vi "FL_Calc_speed_on_the_fly.vi"(1 "Y coord, mm":dbl, 2 "X coord, mm":dbl, 3 "Time per frame, s":dbl) -> (0 "Mouse speed, mm/s":dbl)   [LabVIEW 2016]
doc: "This VI calculates speed using smoothing of the input noisy data according to Holoborodko' algorithm: http://www.holoborodko.com/pavel/numerical-methods/numerical-derivative/smooth-low-noise-differentiator"
uses:
  <vilib>/Analysis/baseanly.llb/Mean (DBL).vi
  <vilib>/Analysis/NI_AALBase.lvlib
panel:
  in  "Speed smoothing type":u16(ring)=3 items=["None", "Holoborodko 2/5", "Holoborodko 2/7", "Holoborodko 2/11", "Holoborodko 4/7"]
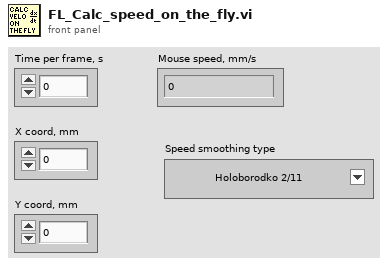
[diagram p1: front panel]
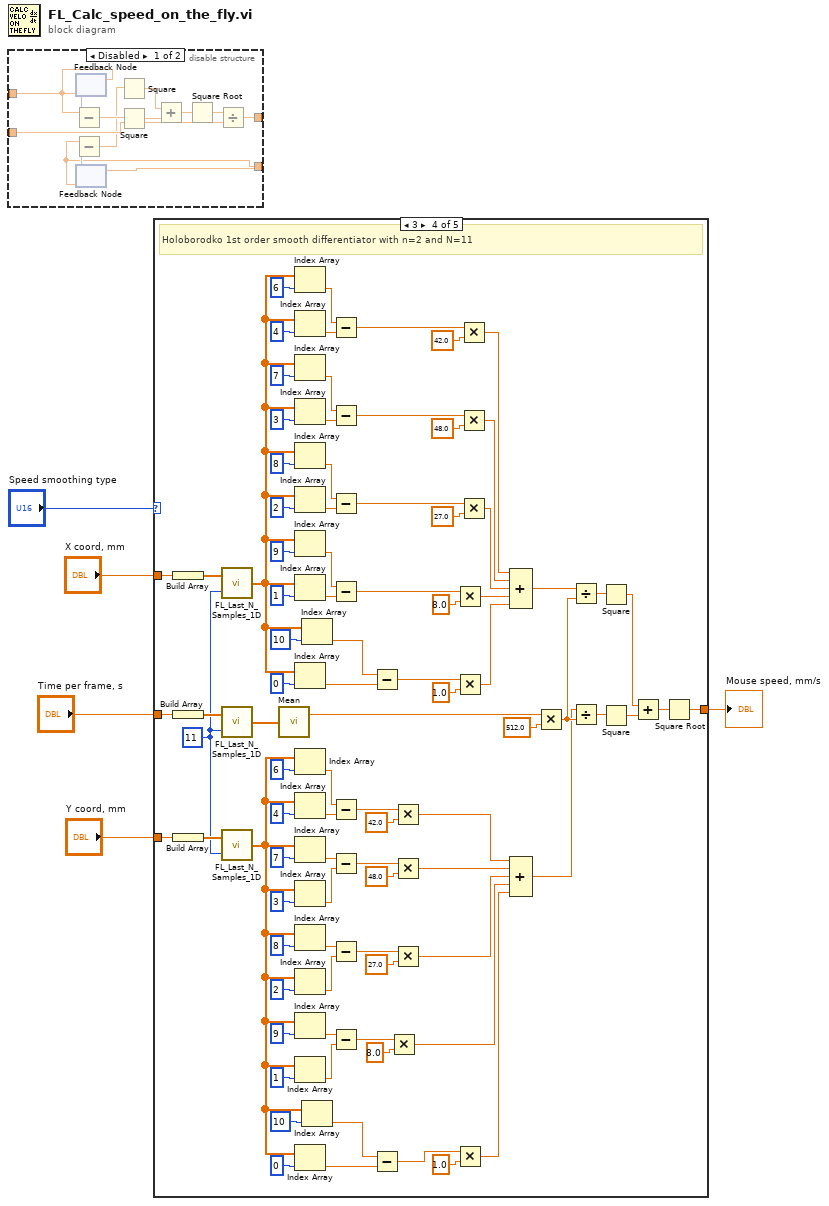
[diagram p0: block diagram]
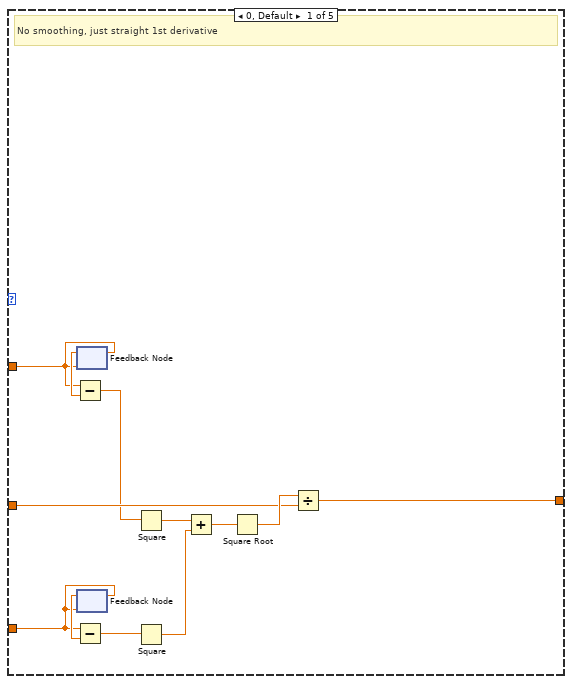
[diagram p2: hidden frame]
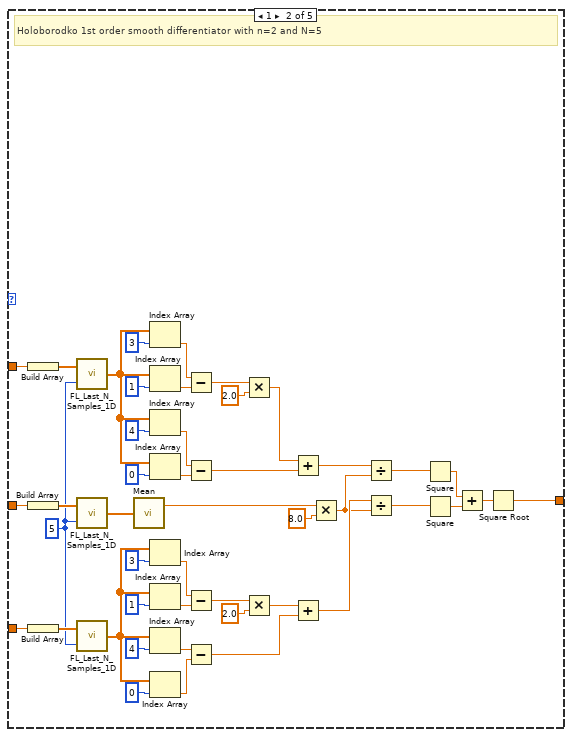
[diagram p3: hidden frame]
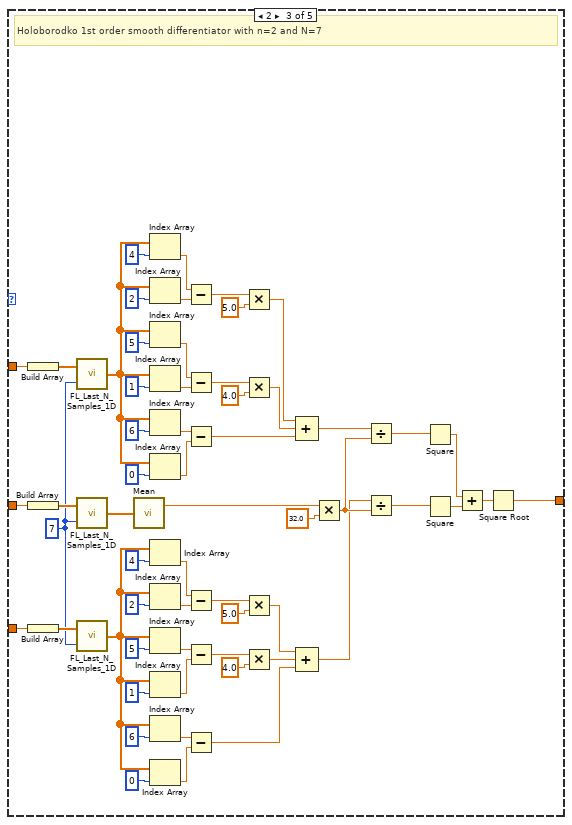
[diagram p4: hidden frame]
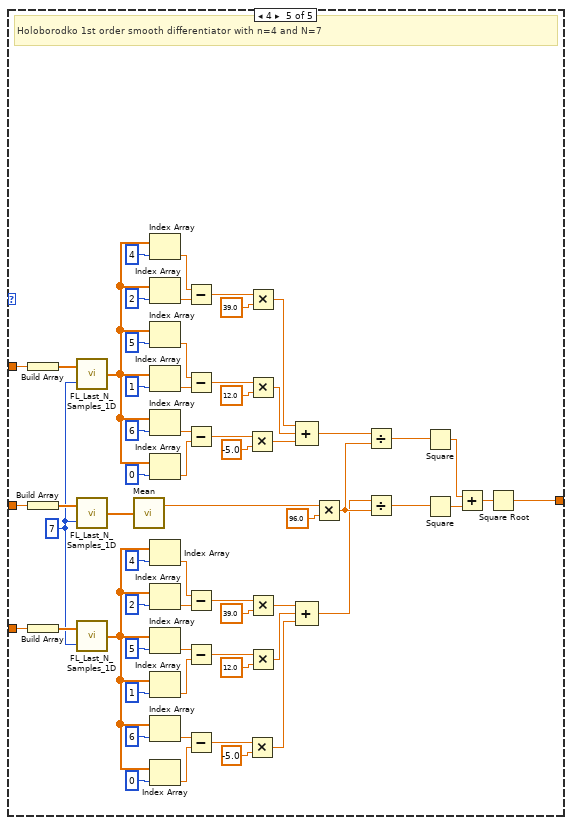
[diagram p5: hidden frame]
diagram:
  n1 = disable-structure shown="Disabled" {
    disable-tunnel: _ -> [w17 _]
    disable-tunnel: [w16 _] -> _
    disable-tunnel: _ -> [w15 _]
    disable-tunnel: _ -> [w6 _]
    frame Disabled {
      n2 = feedback #1(w15) -> (w8)
      n3 = Subtract(x=w15, y=w8) -> (x-y=w10:dbl)
      n4 = feedback-in #1(w15) -> ()
      n5 = feedback #2(w6) -> (w7)
      n6 = Subtract(x=w6, y=w7) -> (x-y=w9:dbl)
      n7 = feedback-in #2(w6) -> ()
      n8 = Square(x=w9) -> (x^2=w12:dbl)
      n9 = Square(x=w10) -> (x^2=w11:dbl)
      n10 = Add(x=w12, y=w11) -> (x+y=w13:dbl)
      n11 = Square Root(x=w13) -> (sqrt(x)=w14:dbl)
      n12 = Divide(x=w14, y=w17) -> (x/y=w16:dbl)
    }
    frame Enabled {
    }
  }
  n13 = case shown="3" "Speed smoothing type" {
    tunnel: "Time per frame, s" -> [w25 w74 w133 w224 w287]
    tunnel: "Y coord, mm" -> [w19 w70 w129 w220 w283]
    tunnel: "X coord, mm" -> [w21 w69 w128 w219 w282]
    tunnel: [w24 w30 w109 w200 w263] -> w2
    frame 0, Default {
      # "No smoothing, just straight 1st derivative"
      n14 = feedback #3(w21) -> (w22:dbl)
      n15 = Subtract(x=w21, y=w22) -> (x-y=w20:dbl)
      n16 = feedback-in #3(w21) -> ()
      n17 = feedback #4(w19) -> (w23:dbl)
      n18 = Subtract(x=w19, y=w23) -> (x-y=w18:dbl)
      n19 = feedback-in #4(w19) -> ()
      n20 = Square(x=w20) -> (x^2=w28:dbl)
      n21 = Square(x=w18) -> (x^2=w29:dbl)
      n22 = Add(x=w28, y=w29) -> (x+y=w27:dbl)
      n23 = Square Root(x=w27) -> (sqrt(x)=w26:dbl)
      n24 = Divide(x=w26, y=w25) -> (x/y=w24:dbl)
    }
    frame 1 {
      w68 = u32 5 ("BufferLengthSamples")
      # "Holoborodko 1st order smooth differentiator with n=2 and N=5"
      n25 = Build Array(w69) -> (w72:dbl[])
      n26 = Build Array(w74) -> (w73:dbl[])
      n27 = Build Array(w70) -> (w71:dbl[])
      n28 = call "FL_Last_N_Samples_1D.vi"("BufferLengthSamples"=w68, "Input Array of strings"=w72) -> ("Output Array of strings"=w58:dbl[])
      n29 = call "FL_Last_N_Samples_1D.vi"("BufferLengthSamples"=w68, "Input Array of strings"=w73) -> ("Output Array of strings"=w67:dbl[])
      n30 = call "FL_Last_N_Samples_1D.vi"("BufferLengthSamples"=w68, "Input Array of strings"=w71) -> ("Output Array of strings"=w37:dbl[])
      n31 = call-poly <vilib>:"Mean.vi"("X"=w67) -> ("mean"=w52:dbl)  [unwired: 1 out]
      n32 = Index Array(array=w58, index=3) -> (element=w64:dbl)
      n33 = Index Array(array=w58, index=1) -> (element=w63:dbl)
      n34 = Index Array(array=w58, index=4) -> (element=w57:dbl)
      n35 = Index Array(array=w58, index=0) -> (element=w56:dbl)
      n36 = Index Array(array=w37, index=3) -> (element=w40:dbl)
      n37 = Index Array(array=w37, index=1) -> (element=w41:dbl)
      n38 = Index Array(array=w37, index=4) -> (element=w46:dbl)
      n39 = Index Array(array=w37, index=0) -> (element=w47:dbl)
      n40 = Subtract(x=w64, y=w63) -> (x-y=w62:dbl)
      n41 = Subtract(x=w57, y=w56) -> (x-y=w54:dbl)
      n42 = Subtract(x=w40, y=w41) -> (x-y=w42:dbl)
      n43 = Subtract(x=w46, y=w47) -> (x-y=w49:dbl)
      n44 = Multiply(x=w62, y=2.0) -> (x*y=w55:dbl)
      n45 = Multiply(x=w42, y=2.0) -> (x*y=w48:dbl)
      n46 = Add(x=w55, y=w54) -> (x+y=w53:dbl)
      n47 = Add(x=w48, y=w49) -> (x+y=w50:dbl)
      n48 = Multiply(x=w52, y=8.0) -> (x*y=w36:dbl)
      n49 = Divide(x=w53, y=w36) -> (x/y=w33:dbl)
      n50 = Divide(x=w50, y=w36) -> (x/y=w31:dbl)
      n51 = Square(x=w33) -> (x^2=w32:dbl)
      n52 = Square(x=w31) -> (x^2=w34:dbl)
      n53 = Add(x=w32, y=w34) -> (x+y=w35:dbl)
      n54 = Square Root(x=w35) -> (sqrt(x)=w30:dbl)
    }
    frame 2 {
      w127 = u32 7 ("BufferLengthSamples")
      # "Holoborodko 1st order smooth differentiator with n=2 and N=7"
      n55 = Build Array(w128) -> (w131:dbl[])
      n56 = Build Array(w133) -> (w132:dbl[])
      n57 = Build Array(w129) -> (w130:dbl[])
      n58 = call "FL_Last_N_Samples_1D.vi"("BufferLengthSamples"=w127, "Input Array of strings"=w131) -> ("Output Array of strings"=w104:dbl[])
      n59 = call "FL_Last_N_Samples_1D.vi"("BufferLengthSamples"=w127, "Input Array of strings"=w132) -> ("Output Array of strings"=w126:dbl[])
      n60 = call "FL_Last_N_Samples_1D.vi"("BufferLengthSamples"=w127, "Input Array of strings"=w130) -> ("Output Array of strings"=w77:dbl[])
      n61 = call-poly <vilib>:"Mean.vi"("X"=w126) -> ("mean"=w117:dbl)  [unwired: 1 out]
      n62 = Index Array(array=w104, index=4) -> (element=w123:dbl)
      n63 = Index Array(array=w104, index=2) -> (element=w122:dbl)
      n64 = Index Array(array=w104, index=5) -> (element=w119:dbl)
      n65 = Index Array(array=w104, index=1) -> (element=w118:dbl)
      n66 = Index Array(array=w104, index=6) -> (element=w107:dbl)
      n67 = Index Array(array=w104, index=0) -> (element=w108:dbl)
      n68 = Index Array(array=w77, index=4) -> (element=w80:dbl)
      n69 = Index Array(array=w77, index=2) -> (element=w81:dbl)
      n70 = Index Array(array=w77, index=5) -> (element=w84:dbl)
      n71 = Index Array(array=w77, index=1) -> (element=w85:dbl)
      n72 = Index Array(array=w77, index=6) -> (element=w87:dbl)
      n73 = Index Array(array=w77, index=0) -> (element=w86:dbl)
      n74 = Subtract(x=w123, y=w122) -> (x-y=w103:dbl)
      n75 = Subtract(x=w119, y=w118) -> (x-y=w101:dbl)
      n76 = Subtract(x=w107, y=w108) -> (x-y=w99:dbl)
      n77 = Subtract(x=w80, y=w81) -> (x-y=w90:dbl)
      n78 = Subtract(x=w84, y=w85) -> (x-y=w92:dbl)
      n79 = Subtract(x=w87, y=w86) -> (x-y=w94:dbl)
      n80 = Multiply(x=w103, y=5.0) -> (x*y=w97:dbl)
      n81 = Multiply(x=w101, y=4.0) -> (x*y=w98:dbl)
      n82 = Multiply(x=w90, y=5.0) -> (x*y=w96:dbl)
      n83 = Multiply(x=w92, y=4.0) -> (x*y=w95:dbl)
      n84 = Compound Arithmetic op=ADD(w97, w98, w99) -> (w76:dbl)
      n85 = Compound Arithmetic op=ADD(w96, w95, w94) -> (w75:dbl)
      n86 = Multiply(x=w117, y=32.0) -> (x*y=w115:dbl)
      n87 = Divide(x=w76, y=w115) -> (x/y=w112:dbl)
      n88 = Divide(x=w75, y=w115) -> (x/y=w110:dbl)
      n89 = Square(x=w112) -> (x^2=w111:dbl)
      n90 = Square(x=w110) -> (x^2=w113:dbl)
      n91 = Add(x=w111, y=w113) -> (x+y=w114:dbl)
      n92 = Square Root(x=w114) -> (sqrt(x)=w109:dbl)
    }
    frame 3 {
      w218 = u32 11 ("BufferLengthSamples")
      # "Holoborodko 1st order smooth differentiator with n=2 and N=11"
      n93 = Build Array(w219) -> (w222:dbl[])
      n94 = Build Array(w224) -> (w223:dbl[])
      n95 = Build Array(w220) -> (w221:dbl[])
      n96 = call "FL_Last_N_Samples_1D.vi"("BufferLengthSamples"=w218, "Input Array of strings"=w222) -> ("Output Array of strings"=w173:dbl[])
      n97 = call "FL_Last_N_Samples_1D.vi"("BufferLengthSamples"=w218, "Input Array of strings"=w223) -> ("Output Array of strings"=w217:dbl[])
      n98 = call "FL_Last_N_Samples_1D.vi"("BufferLengthSamples"=w218, "Input Array of strings"=w221) -> ("Output Array of strings"=w135:dbl[])
      n99 = call-poly <vilib>:"Mean.vi"("X"=w217) -> ("mean"=w208:dbl)  [unwired: 1 out]
      n100 = Index Array(array=w173, index=6) -> (element=w214:dbl)
      n101 = Index Array(array=w173, index=4) -> (element=w213:dbl)
      n102 = Index Array(array=w173, index=7) -> (element=w210:dbl)
      n103 = Index Array(array=w173, index=3) -> (element=w209:dbl)
      n104 = Index Array(array=w173, index=8) -> (element=w198:dbl)
      n105 = Index Array(array=w173, index=2) -> (element=w199:dbl)
      n106 = Index Array(array=w173, index=9) -> (element=w181:dbl)
      n107 = Index Array(array=w173, index=1) -> (element=w180:dbl)
      n108 = Index Array(array=w173, index=0) -> (element=w179:dbl)
      n109 = Index Array(array=w135, index=6) -> (element=w138:dbl)
      n110 = Index Array(array=w135, index=4) -> (element=w139:dbl)
      n111 = Index Array(array=w135, index=7) -> (element=w142:dbl)
      n112 = Index Array(array=w135, index=3) -> (element=w143:dbl)
      n113 = Index Array(array=w135, index=8) -> (element=w145:dbl)
      n114 = Index Array(array=w135, index=2) -> (element=w144:dbl)
      n115 = Index Array(array=w135, index=9) -> (element=w161:dbl)
      n116 = Index Array(array=w135, index=1) -> (element=w162:dbl)
      n117 = Index Array(array=w135, index=0) -> (element=w163:dbl)
      n118 = Index Array(array=w173, index=10) -> (element=w178:dbl)
      n119 = Index Array(array=w135, index=10) -> (element=w164:dbl)
      n120 = Subtract(x=w214, y=w213) -> (x-y=w195:dbl)
      n121 = Subtract(x=w210, y=w209) -> (x-y=w193:dbl)
      n122 = Subtract(x=w198, y=w199) -> (x-y=w191:dbl)
      n123 = Subtract(x=w181, y=w180) -> (x-y=w184:dbl)
      n124 = Subtract(x=w138, y=w139) -> (x-y=w148:dbl)
      n125 = Subtract(x=w142, y=w143) -> (x-y=w150:dbl)
      n126 = Subtract(x=w145, y=w144) -> (x-y=w152:dbl)
      n127 = Subtract(x=w161, y=w162) -> (x-y=w158:dbl)
      n128 = Subtract(x=w178, y=w179) -> (x-y=w175:dbl)
      n129 = Subtract(x=w164, y=w163) -> (x-y=w167:dbl)
      n130 = Multiply(x=w158, y=8.0) -> (x*y=w169:dbl)
      n131 = Multiply(x=w148, y=42.0) -> (x*y=w154:dbl)
      n132 = Multiply(x=w150, y=48.0) -> (x*y=w153:dbl)
      n133 = Multiply(x=w152, y=27.0) -> (x*y=w155:dbl)
      n134 = Multiply(x=w184, y=8.0) -> (x*y=w172:dbl)
      n135 = Multiply(x=w175, y=1.0) -> (x*y=w171:dbl)
      n136 = Multiply(x=w167, y=1.0) -> (x*y=w170:dbl)
      n137 = Multiply(x=w195, y=42.0) -> (x*y=w189:dbl)
      n138 = Multiply(x=w193, y=48.0) -> (x*y=w190:dbl)
      n139 = Multiply(x=w191, y=27.0) -> (x*y=w187:dbl)
      n140 = Compound Arithmetic op=ADD(w189, w190, w187, w172, w171) -> (w188:dbl)
      n141 = Compound Arithmetic op=ADD(w154, w153, w155, w169, w170) -> (w134:dbl)
      n142 = Multiply(x=w208, y=512.0) -> (x*y=w206:dbl)
      n143 = Divide(x=w188, y=w206) -> (x/y=w203:dbl)
      n144 = Divide(x=w134, y=w206) -> (x/y=w201:dbl)
      n145 = Square(x=w203) -> (x^2=w202:dbl)
      n146 = Square(x=w201) -> (x^2=w204:dbl)
      n147 = Add(x=w202, y=w204) -> (x+y=w205:dbl)
      n148 = Square Root(x=w205) -> (sqrt(x)=w200:dbl)
    }
    frame 4 {
      w281 = u32 7 ("BufferLengthSamples")
      # "Holoborodko 1st order smooth differentiator with n=4 and N=7"
      n149 = Build Array(w282) -> (w285:dbl[])
      n150 = Build Array(w287) -> (w286:dbl[])
      n151 = Build Array(w283) -> (w284:dbl[])
      n152 = call "FL_Last_N_Samples_1D.vi"("BufferLengthSamples"=w281, "Input Array of strings"=w285) -> ("Output Array of strings"=w258:dbl[])
      n153 = call "FL_Last_N_Samples_1D.vi"("BufferLengthSamples"=w281, "Input Array of strings"=w286) -> ("Output Array of strings"=w280:dbl[])
      n154 = call "FL_Last_N_Samples_1D.vi"("BufferLengthSamples"=w281, "Input Array of strings"=w284) -> ("Output Array of strings"=w231:dbl[])
      n155 = call-poly <vilib>:"Mean.vi"("X"=w280) -> ("mean"=w271:dbl)  [unwired: 1 out]
      n156 = Index Array(array=w258, index=4) -> (element=w277:dbl)
      n157 = Index Array(array=w258, index=2) -> (element=w276:dbl)
      n158 = Index Array(array=w258, index=5) -> (element=w273:dbl)
      n159 = Index Array(array=w258, index=1) -> (element=w272:dbl)
      n160 = Index Array(array=w258, index=6) -> (element=w261:dbl)
      n161 = Index Array(array=w258, index=0) -> (element=w262:dbl)
      n162 = Index Array(array=w231, index=4) -> (element=w234:dbl)
      n163 = Index Array(array=w231, index=2) -> (element=w235:dbl)
      n164 = Index Array(array=w231, index=5) -> (element=w238:dbl)
      n165 = Index Array(array=w231, index=1) -> (element=w239:dbl)
      n166 = Index Array(array=w231, index=6) -> (element=w241:dbl)
      n167 = Index Array(array=w231, index=0) -> (element=w240:dbl)
      n168 = Subtract(x=w277, y=w276) -> (x-y=w257:dbl)
      n169 = Subtract(x=w273, y=w272) -> (x-y=w255:dbl)
      n170 = Subtract(x=w261, y=w262) -> (x-y=w253:dbl)
      n171 = Subtract(x=w234, y=w235) -> (x-y=w244:dbl)
      n172 = Subtract(x=w238, y=w239) -> (x-y=w246:dbl)
      n173 = Subtract(x=w241, y=w240) -> (x-y=w248:dbl)
      n174 = Multiply(x=w253, y=-5.0) -> (x*y=w228:dbl)
      n175 = Multiply(x=w248, y=-5.0) -> (x*y=w226:dbl)
      n176 = Multiply(x=w257, y=39.0) -> (x*y=w251:dbl)
      n177 = Multiply(x=w255, y=12.0) -> (x*y=w252:dbl)
      n178 = Multiply(x=w244, y=39.0) -> (x*y=w250:dbl)
      n179 = Multiply(x=w246, y=12.0) -> (x*y=w249:dbl)
      n180 = Compound Arithmetic op=ADD(w251, w252, w228) -> (w230:dbl)
      n181 = Compound Arithmetic op=ADD(w250, w249, w226) -> (w229:dbl)
      n182 = Multiply(x=w271, y=96.0) -> (x*y=w269:dbl)
      n183 = Divide(x=w230, y=w269) -> (x/y=w266:dbl)
      n184 = Divide(x=w229, y=w269) -> (x/y=w264:dbl)
      n185 = Square(x=w266) -> (x^2=w265:dbl)
      n186 = Square(x=w264) -> (x^2=w267:dbl)
      n187 = Add(x=w265, y=w267) -> (x+y=w268:dbl)
      n188 = Square Root(x=w268) -> (sqrt(x)=w263:dbl)
    }
  }
  "Mouse speed, mm/s" <- w2
